vi "OCR_Build Body rectangles.vi"(8 "Error":errorcluster, 9 "Text Location":T3, 10 "Color Array":T2[](array[typedef]), 11 "2D Image":T1) -> (0 "Error Out":errorcluster, 3 "Body Rect Array Out":T4[](array[typedef]))   [LabVIEW 2009]
doc: "Seperates the icon body bounds into an array of each line in the body."
uses:
  Controls/Cluster/Cluster_Text Rect.ctl
  Controls/Cluster/Cluster_Region info.ctl
  Controls/Cluster/Cluster_Top Left position.ctl
  Controls/Cluster/Cluster_Text Color Set.ctl
  Controls/Cluster/Cluster_Line Location and status.ctl
  Controls/Array/Color Box Array_2D Icon Viewer.ctl
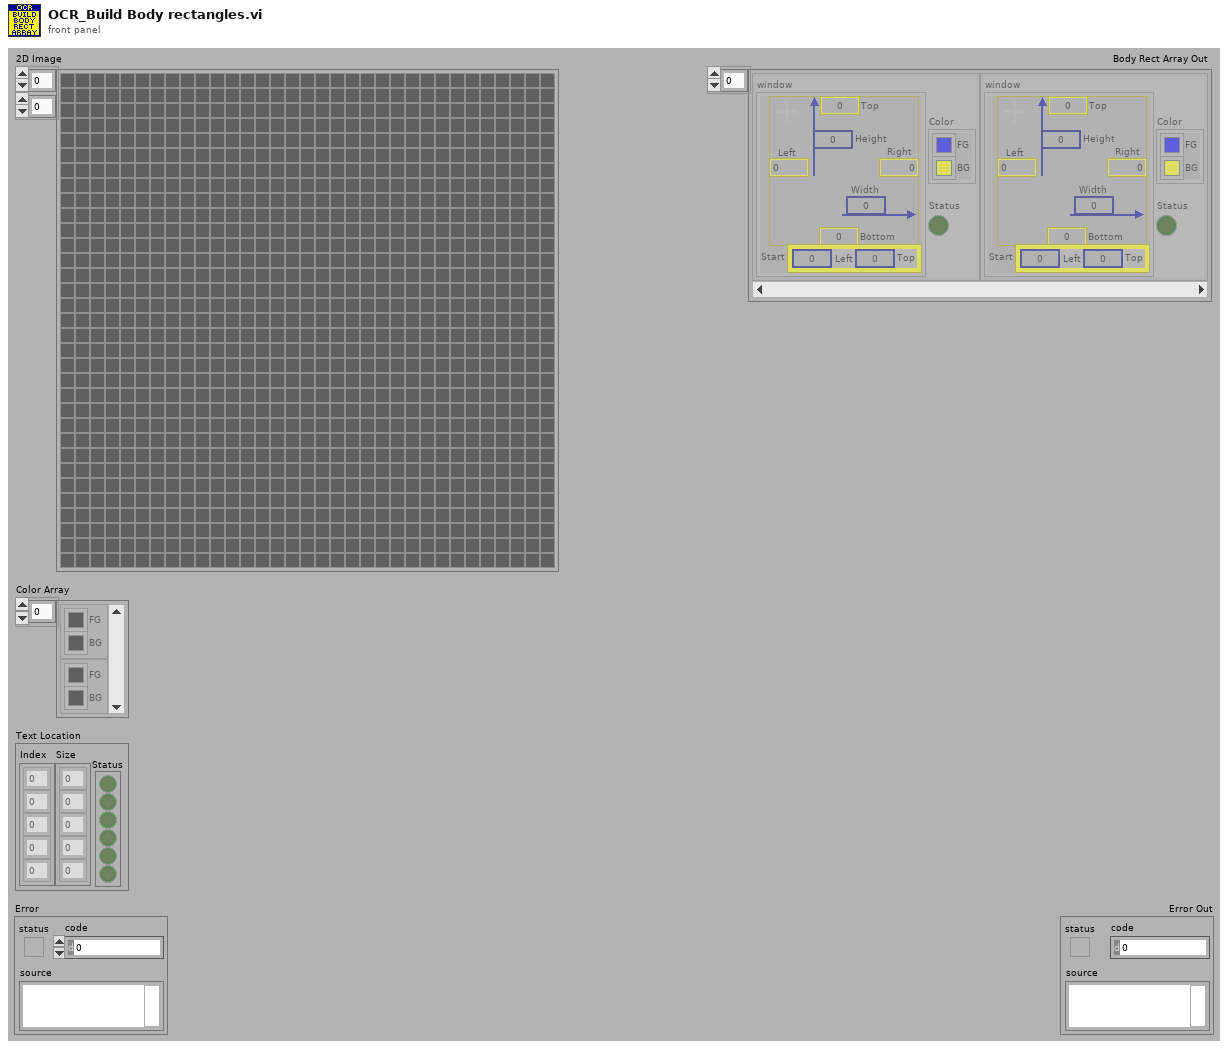
[diagram p1: front panel]
types:
  T1 = typedef "Color Box Array_2D Icon Viewer.ctl" = u32[][]
  T2 = typedef "Cluster_Text Color Set.ctl" = cluster{"BG":u32, "FG":u32}
  T3 = typedef "Cluster_Line Location and status.ctl" = cluster{"Index":i16[], "Status":bool[], "Size":i32[]}
  T4 = typedef "Cluster_Text Rect.ctl" = cluster{"window":T5, "Color":T2, "Status":bool}
  T5 = typedef "Cluster_Region info.ctl" = cluster{"Left":i32, "Top":i32, "Right":i32, "Bottom":i32, "Width":u32, "Height":u32, "Start":T6}
  T6 = typedef "Cluster_Top Left position.ctl" = cluster{"Left":i32, "Top":i32}
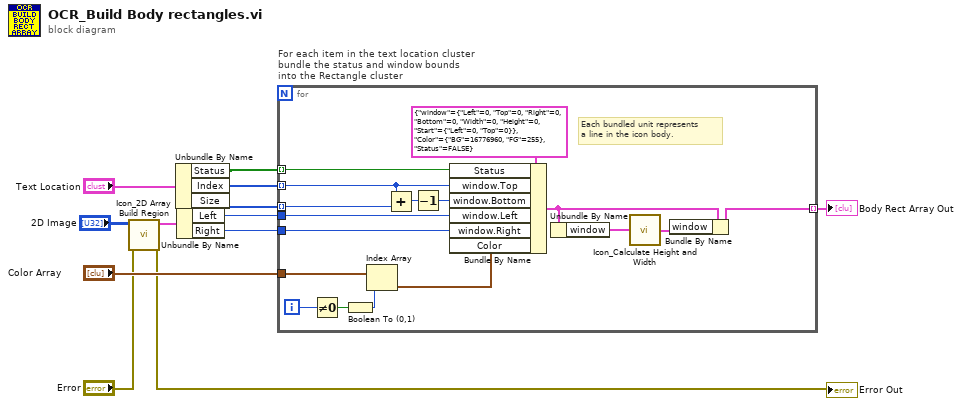
[diagram p0: block diagram]
diagram:
  n1 = call "Icon_2D Array Build Region.vi"("Error"="Error", "2D Image"="2D Image") -> ("Error Out"=→"Error Out":errorcluster, "Region Out"=w3:T5)  [unwired: 7 in, 1 out]
  n2 = Unbundle By Name("Text Location") -> ("Status"=w9:bool[], "Index"=w10:i16[], "Size"=w8:i32[])
  n3 = Unbundle By Name(w3) -> ("Left"=w7:i32, "Right"=w6:i32)
  n4 = for "For each item in the text location cluster\nbundle the status and window bounds\ninto the Rectangle cluster" {
    tunnel: w10 -> [w29] mode=indexing
    tunnel: [w23] -> w12 mode=indexing
    tunnel: w9 -> [w27] mode=indexing
    tunnel: w8 -> [w26] mode=indexing
    tunnel: w7 -> [w20]
    tunnel: w6 -> [w19]
    tunnel: "Color Array" -> [w15]
    i -> [w17]
    # "Each bundled unit represents\na line in the icon body."
    n5 = Not Equal To 0?(x=w17) -> (x != 0?=w16:bool)
    n6 = Boolean To (0,1)(Boolean=w16) -> (0, 1=w14:i16)
    n7 = Index Array(array=w15, index=w14) -> (element=w13:T2)
    n8 = Add(x=w29, y=w26) -> (x+y=w28:i32)
    n9 = Decrement(x=w28) -> (x-1=w21:i32)
    n10 = Bundle By Name(cluster=T4 {"window"={"Left"=0, "Top"=0, "Right"=0, "Bottom"=0, "Width"=0, "Height"=0, "Start"={"Left"=0, "Top"=0}}, "Color"={"BG"=16776960, "FG"=255}, "Status"=FALSE} ("Body Rect"), "Status"=w27, "window.Top"=w29, "window.Bottom"=w21, "window.Left"=w20, "window.Right"=w19, "Color"=w13) -> (w24:T4)
    n11 = Unbundle By Name(w24) -> ("window"=w25:T5)
    n12 = call "Icon_Calculate Height and Width.vi"("Region"=w25) -> ("Region Out"=w22:T5)  [unwired: 4 in]
    n13 = Bundle By Name(cluster=w24, "window"=w22) -> (w23:T4)
  }
  "Body Rect Array Out" <- w12
